vi "Initalize OPC UA.vi"(8 "error in (no error)":errorcluster, 11 "SM EOL Station Actor in":refnum<class "PLC Sim Controller Actor.lvclass">) -> (0 "error out":errorcluster, 3 "SM EOL Station Actor out":refnum<class "PLC Sim Controller Actor.lvclass">)   [LabVIEW 2019, in "PLC Sim Controller Actor.lvlib" / "PLC Sim Controller Actor.lvclass"]
uses:
  PLC Sim Controller Actor.lvclass
  <vilib>/OPCUA/controls/Supported Security Policies.ctl
  PLC Sim Controller Actor.lvclass/PLC Sim Controller Actor.ctl
  <vilib>/OPCUA/NI OPC UA Server.lvlib
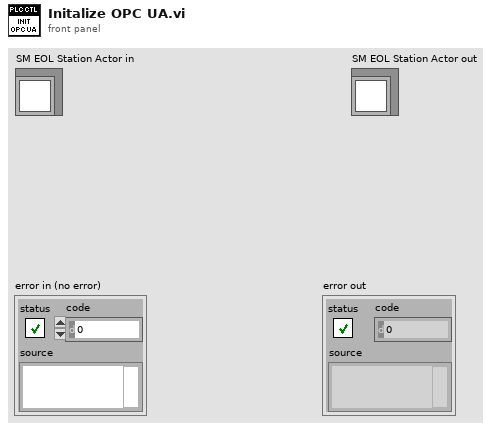
[diagram p1: front panel]
types:
  T1 = typedef "Supported Security Policies.ctl" = cluster{"None":bool, "Sign with Basic128Rsa15":bool, "Sign and Encrypt with Basic128Rsa15":bool, "Sign with Basic256":bool, "Sign and Encrypt with Basic256":bool}
  T2 = typedef "OPC UA Server Refnum.ctl" = refnum<k21>
  T3 = typedef "NodeId.ctl" = string
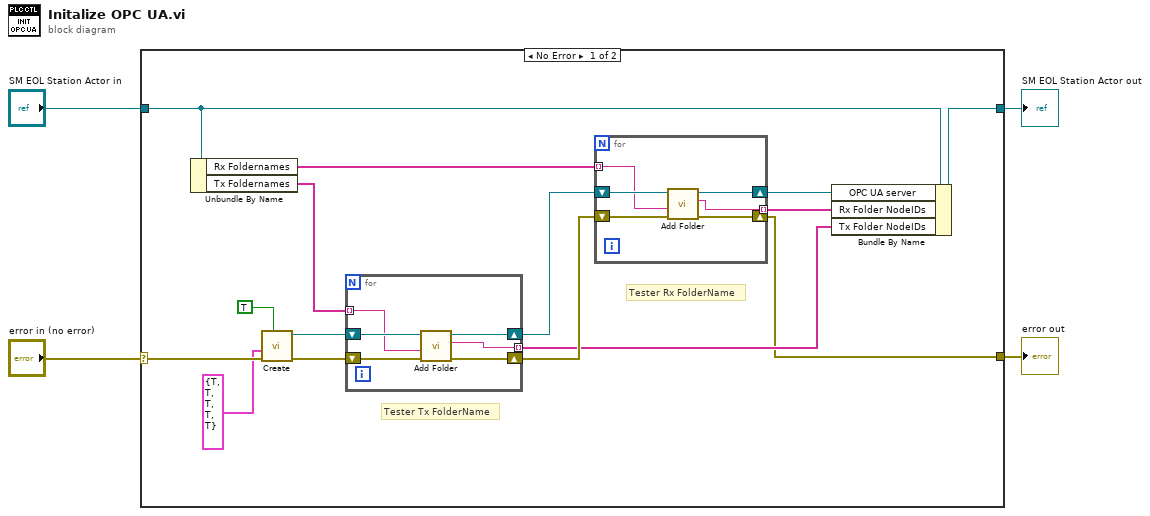
[diagram p0: block diagram]
diagram:
  n1 = case shown="No Error" "error in (no error)" {
    selector: "error in (no error)" -> [w19 w33]
    tunnel: [w5 w33] -> w3
    tunnel: [w9 w32] -> w1
    tunnel: "SM EOL Station Actor in" -> [w10 w32]
    frame No Error {
      # "Tester Rx FolderName"
      # "Tester Tx FolderName"
      n2 = Unbundle By Name(w10) -> ("Rx Foldernames"=w13:string[], "Tx Foldernames"=w12:string[])
      n3 = call <vilib>:"Create.vi"("trust all clients (F)"=TRUE, "error in (no error)"=w19, "supported security policies (None)"=T1 {"None"=TRUE, "Sign with Basic128Rsa15"=TRUE, "Sign and Encrypt with Basic128Rsa15"=TRUE, "Sign with Basic256"=TRUE, "Sign and Encrypt with Basic256"=TRUE}) -> ("error out"=w16:errorcluster, "OPC UA server refnum out"=w15:T2)  [unwired: 6 in, 1 out]
      n4 = for {
        shift-right: [w30] -> w11
        shift-left: w16 -> [w31]
        shift-right: [w28] -> w14
        shift-left: w15 -> [w29]
        tunnel: w12 -> [w27] mode=indexing
        tunnel: [w26] -> w6 mode=indexing
        n5 = call <vilib>:"Add Folder.vi"("error in (no error)"=w31, "folder name"=w27, "OPC UA server refnum in"=w29) -> ("error out"=w30:errorcluster, "folder node ID"=w26:T3, "OPC UA server refnum out"=w28:T2)  [unwired: 5 in]
      }
      n6 = for {
        tunnel: [w24] -> w7 mode=indexing
        shift-right: [w23] -> w8
        shift-left: w14 -> [w25]
        tunnel: w13 -> [w22] mode=indexing
        shift-right: [w20] -> w5
        shift-left: w11 -> [w21]
        n7 = call <vilib>:"Add Folder.vi"("error in (no error)"=w21, "folder name"=w22, "OPC UA server refnum in"=w25) -> ("error out"=w20:errorcluster, "folder node ID"=w24:T3, "OPC UA server refnum out"=w23:T2)  [unwired: 5 in]
      }
      n8 = Bundle By Name(cluster=w10, "OPC UA server"=w8, "Rx Folder NodeIDs"=w7, "Tx Folder NodeIDs"=w6) -> (w9:refnum<class "PLC Sim Controller Actor.lvclass">)
    }
    frame Error {
    }
  }
  "error out" <- w3
  "SM EOL Station Actor out" <- w1
